vi "timer1.vi"(8 "error in (no error)":errorcluster, 11 "Action":T1) -> (0 "error out":errorcluster, 3 "Numeric":dbl)   [LabVIEW 2023]
uses:
  #typedef_action.ctl
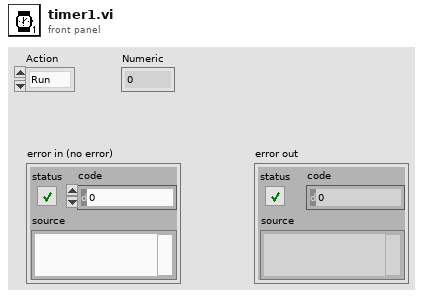
[diagram p1: front panel]
types:
  T1 = typedef "#typedef_action.ctl" = enum16{"Run", "Reset"}
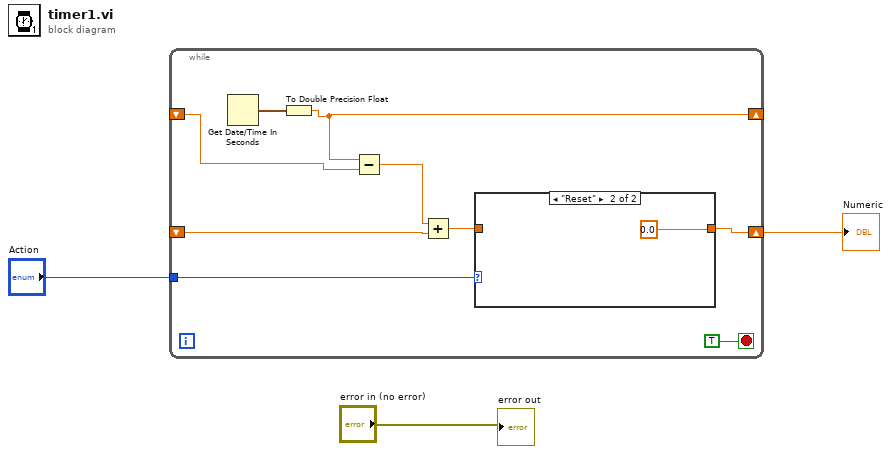
[diagram p0: block diagram]
diagram:
  n1 = while {
    shift-right: [w5] -> _
    shift-left: _ -> [w4]
    shift-right: [w8] -> w3
    shift-left: _ -> [w10]
    tunnel: "Action" -> [w9]
    stop <- TRUE stop-if-true
    n2 = Get Date/Time In Seconds() -> (seconds since 1Jan1904=w12:timestamp)
    n3 = To Double Precision Float(number=w12) -> (double precision float=w5:dbl)
    n4 = Subtract(x=w5, y=w4) -> (x-y=w11:dbl)
    n5 = Add(x=w11, y=w10) -> (x+y=w7:dbl)
    n6 = case shown="\"Reset\"" w9 {
      tunnel: [w13 0.0] -> w8
      tunnel: w7 -> [w13 _]
      frame "Run", Default {
      }
      frame "Reset" {
      }
    }
  }
  "Numeric" <- w3
  "error out" <- "error in (no error)"
